vi "Actor Core.vi"(8 "error in":errorcluster caption="错误输入", 11 "DialogueM in":refnum<class "DialogueM.lvclass"> caption="操作者输入") -> (0 "error out":errorcluster caption="错误输出", 3 "Actor out":refnum<class "Actor.lvclass"> caption="操作者输出")   [LabVIEW 2014, in "DialogueManagement.lvlib" / "DialogueM.lvclass"]
doc: "(<B>文件名</B>：Actor Framework.lvlib:Actor.lvclass:Actor Core.vi)\n\n接收发送至操作者的消息，响应消息并处理可能导致操作者关闭的错误。\n\n子孙类重写该VI，使操作者完成特定的任务。使用调用父方法节点实现重写。"
uses:
  DialogueM.lvclass
  <vilib>/ActorFramework/Actor/Actor.lvclass
  <vilib>/ActorFramework/Actor/Actor.lvclass/Actor.ctl
  DialogueM.lvclass/DialogueM.ctl
  <vilib>/ActorFramework/Message Enqueuer/Message Enqueuer.lvclass/Message Enqueuer.ctl
  <vilib>/ActorFramework/Message Enqueuer/Enqueue.vi
  <vilib>/ActorFramework/Message Priority Queue/Priority Enqueue.vi
panel:
  out "Actor out 2":refnum<class "Actor.lvclass"> caption="操作者输出"
  out "语音信号输出字符串 2":string
  in  "停止信号":bool
  out "系统回应 4":string caption="标准输出"
  out "CM #":i32=-1
  out "InstructionIn":string
  out "系统回应 3":string caption="标准输出"
  out "系统回应 2":string caption="标准输出"
  out "格式化机器人指令":string[][](array[string])
  out "系统回应":string caption="标准输出"
  in  "重来":bool
  out "显示窗口":string
  out "语音信号输出字符串":string
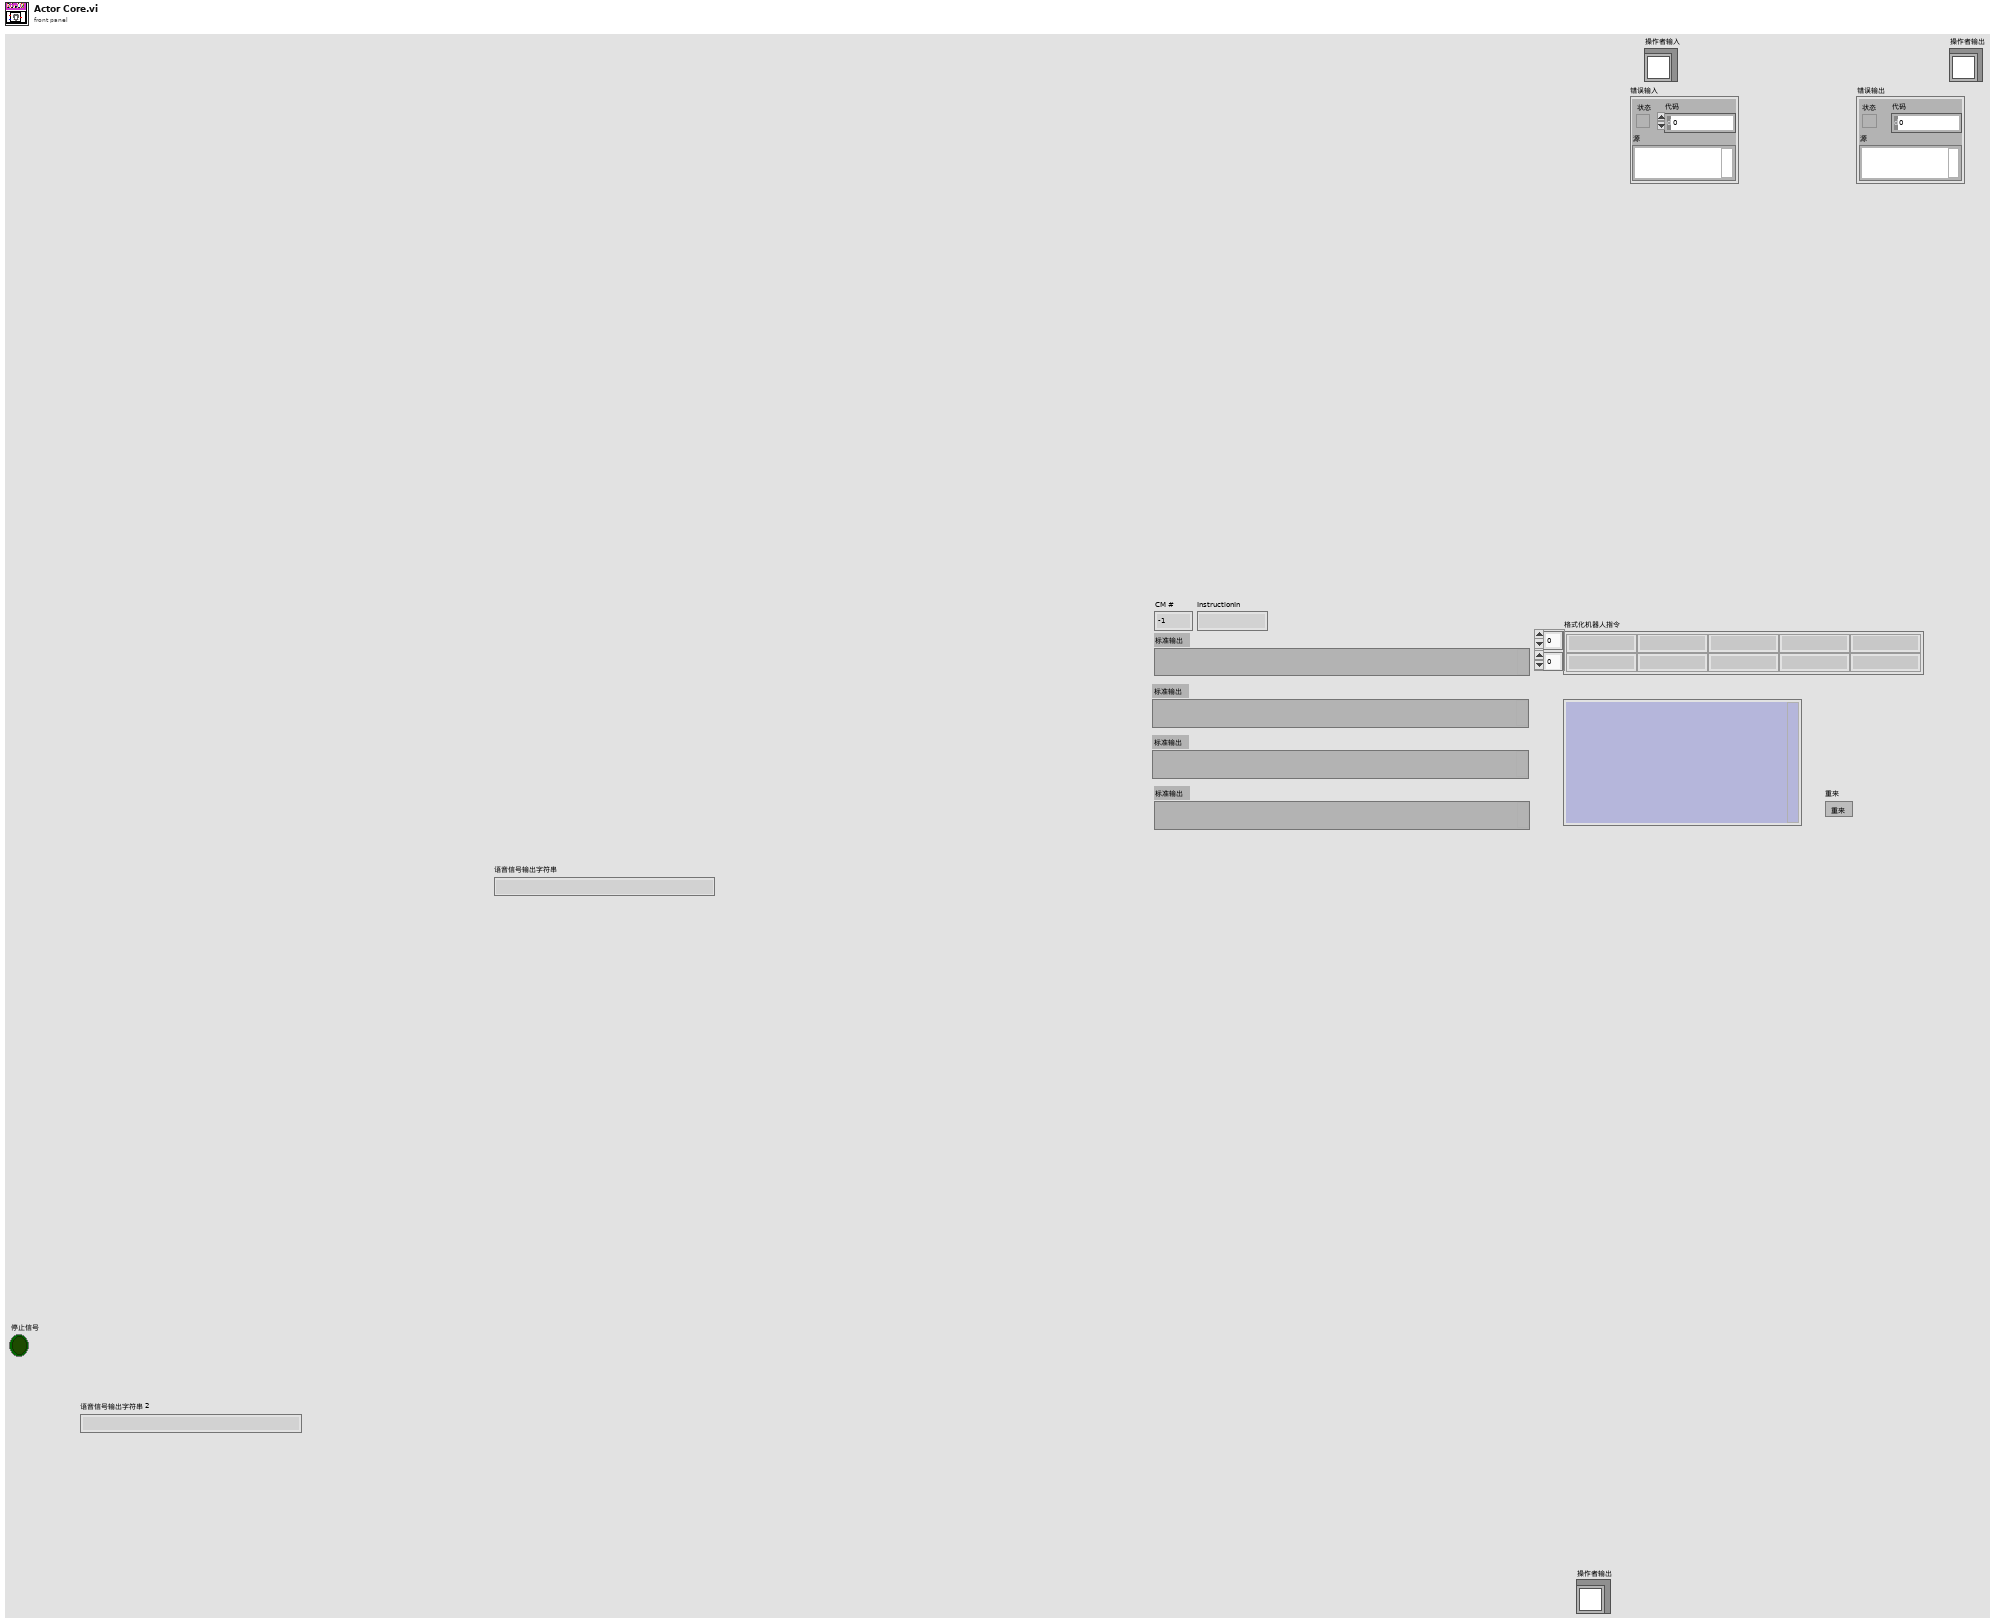
[diagram p1: front panel]
types:
  T1 = cluster{"输出数组":string[][], "CM #":i32, i32, string}
  T2 = cluster{"Stop":refnum<user-event>, "Text":refnum<user-event>, "Connected":refnum<user-event>}
  T3 = enum16{"open", "replace", "create", "open or create", "replace or create", "replace or create with confirmation"}
  T4 = cluster{"输出数组":string[][], "CM #":i32, "CM #":i32, string}
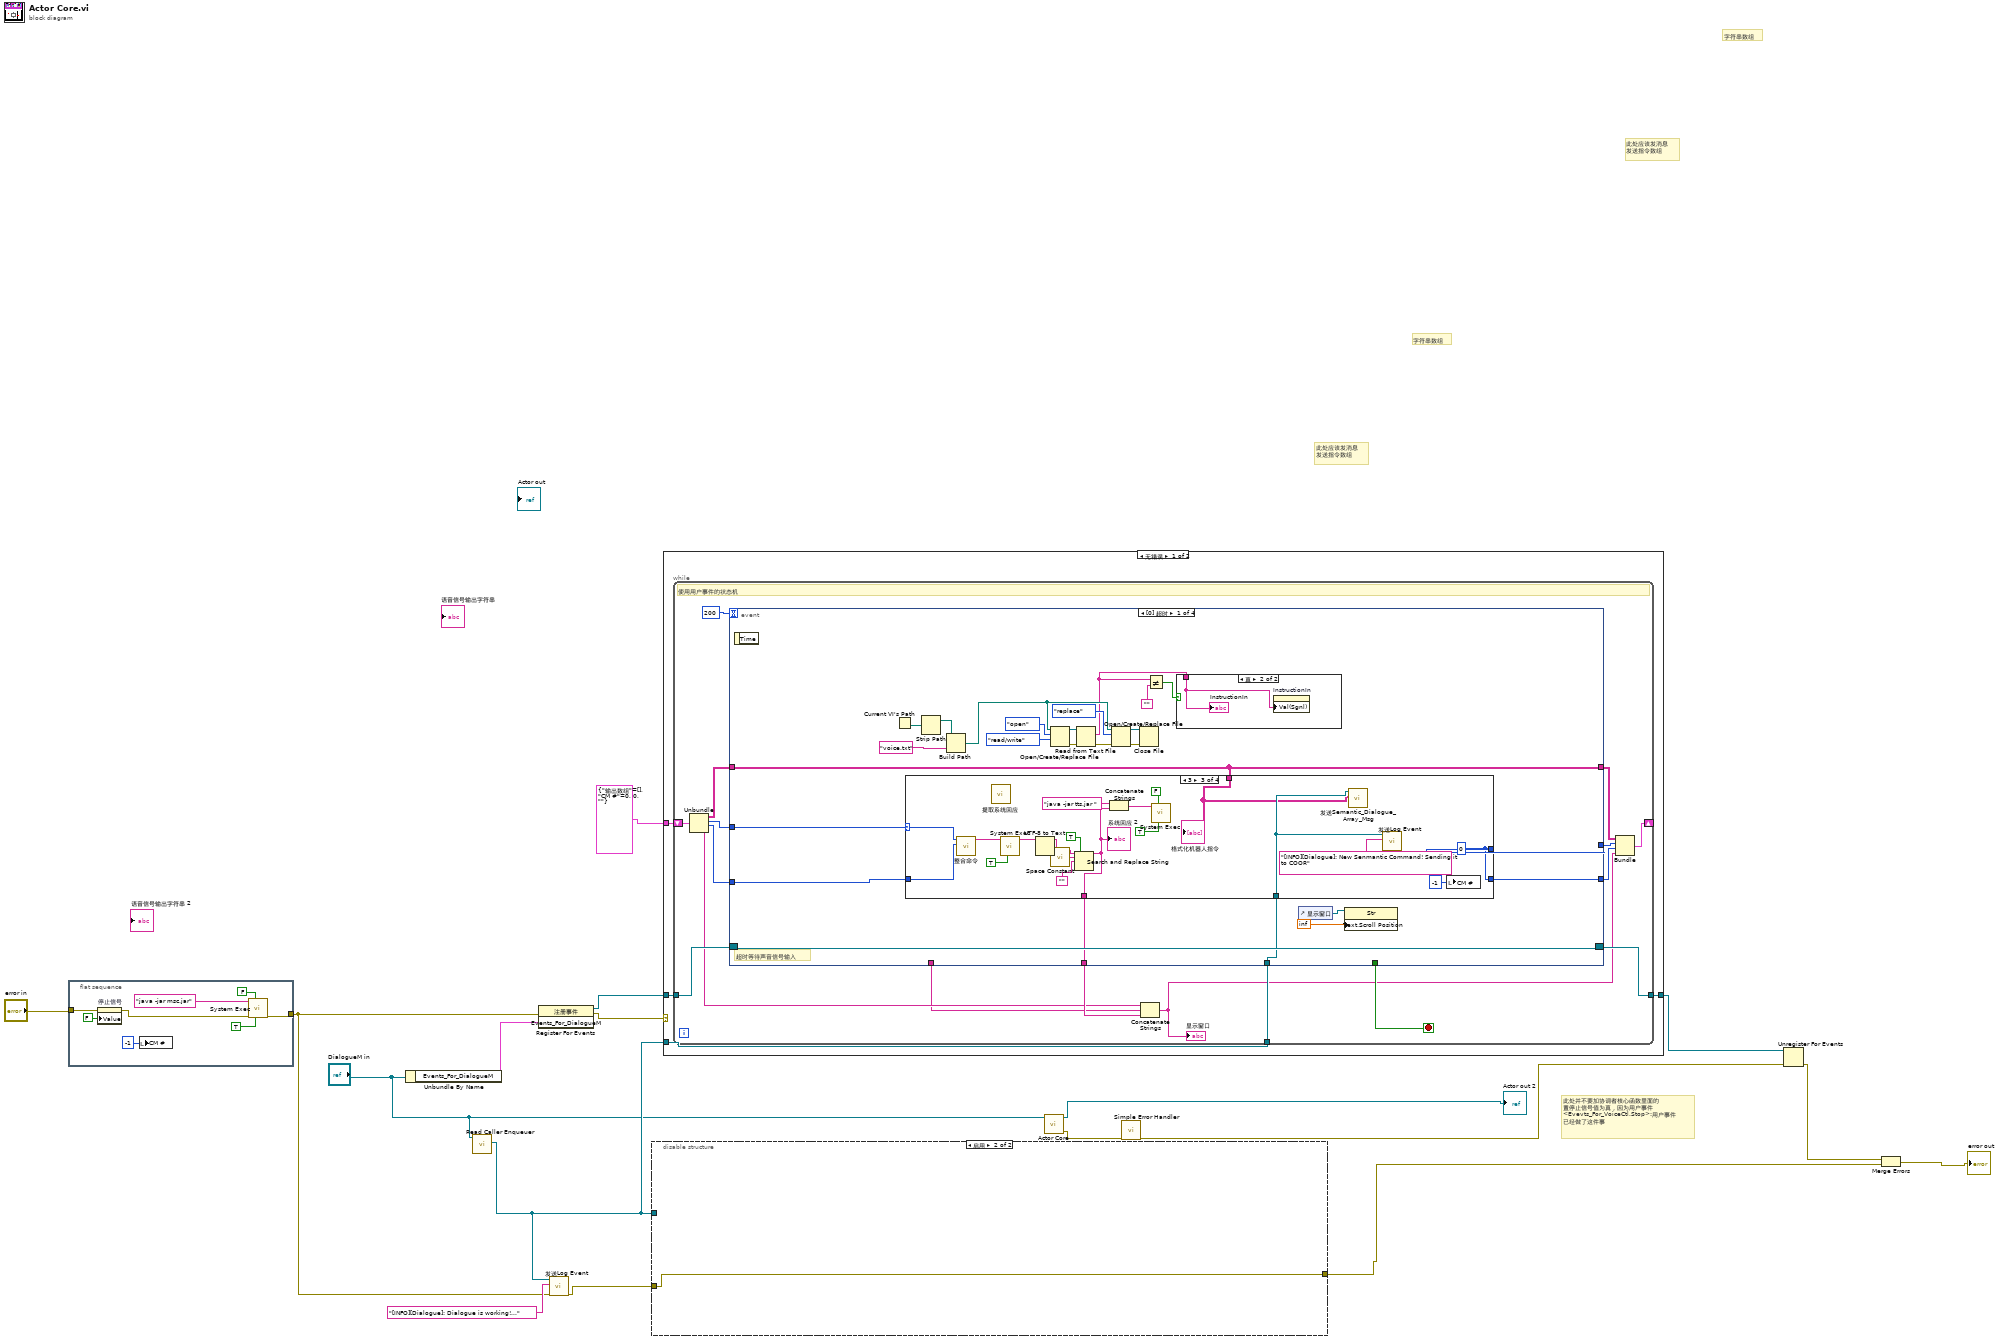
[diagram p0: block diagram]
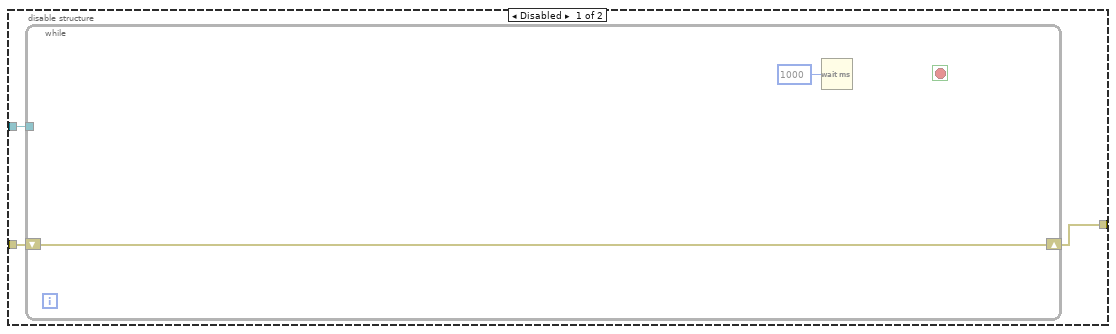
[diagram p2: hidden frame]
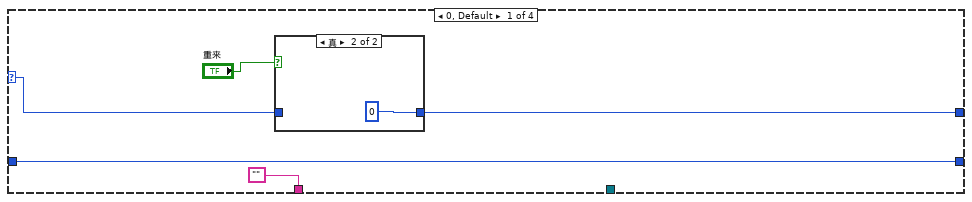
[diagram p3: hidden frame]
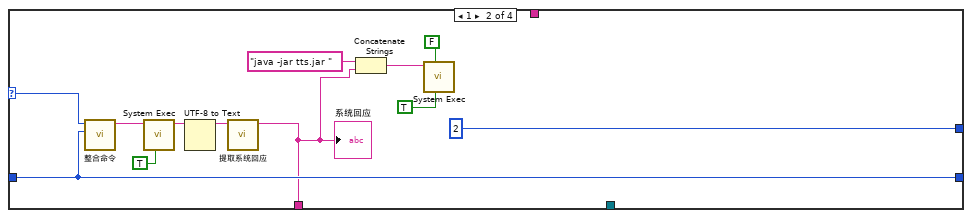
[diagram p5: hidden frame]
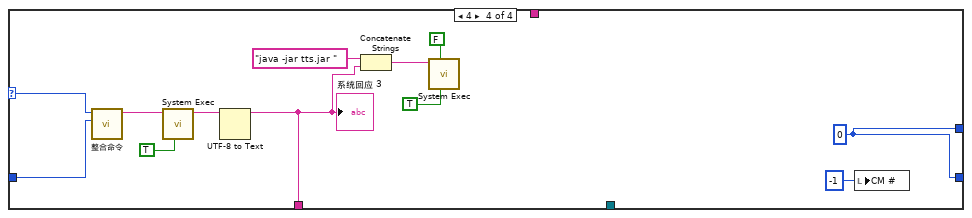
[diagram p6: hidden frame]
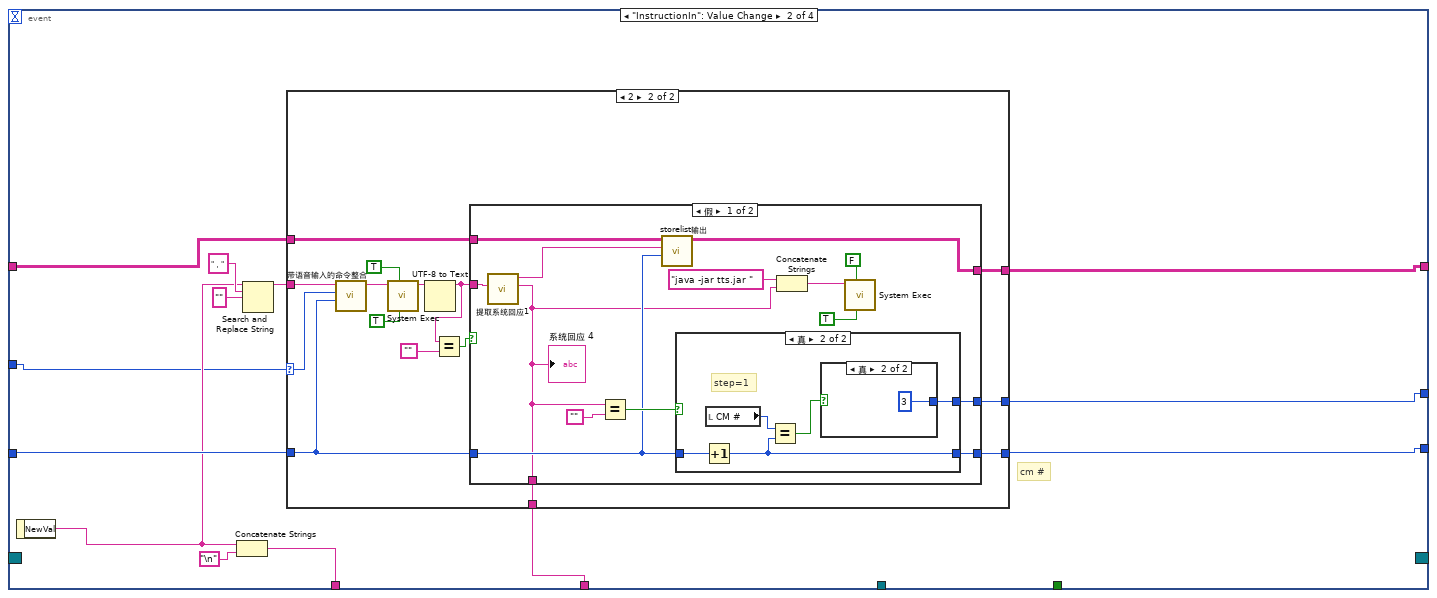
[diagram p8: hidden frame]
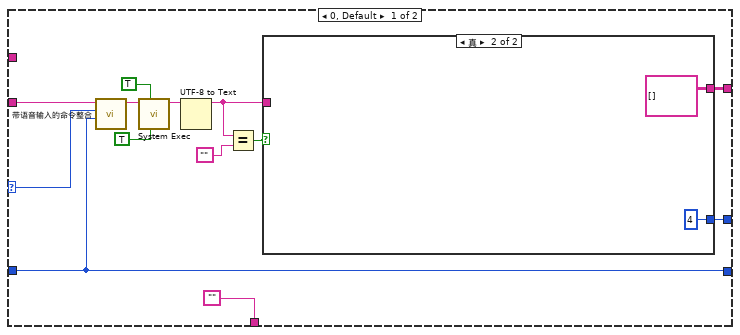
[diagram p9: hidden frame]
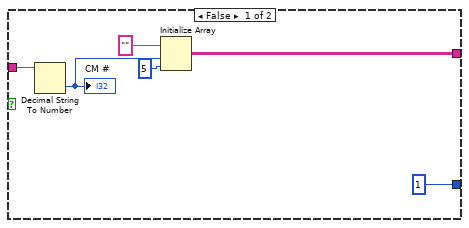
[diagram p10: hidden frame]
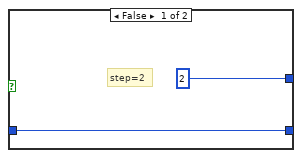
[diagram p11: hidden frame]
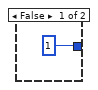
[diagram p12: hidden frame]
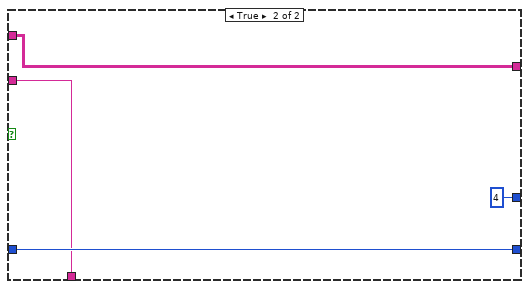
[diagram p13: hidden frame]
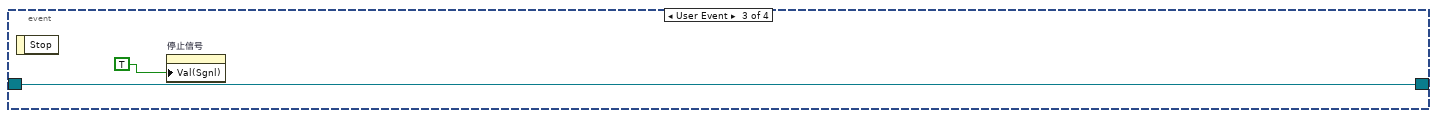
[diagram p14: hidden frame]
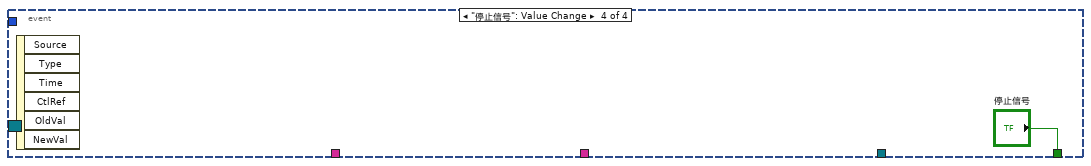
[diagram p15: hidden frame]
diagram:
  # "字符串数组"
  # "此处应该发消息\n发送指令数组"
  # "此处并不要加协调者核心函数里面的\n置停止信号值为真，因为用户事件\n<Evevts_For_VoiceCtl.Stop>:用户事件\n已经做了这件事"
  # "字符串数组"
  # "此处应该发消息\n发送指令数组"
  n1 = flat-sequence {
    tunnel: "error in" -> [w25]
    tunnel: [w19] -> w6
    frame #0 {
      n2 = property on="停止信号" class="Bool (严格)"(error in=w25, "Value"=FALSE ("停止信号")) -> (error out=w20:errorcluster)  [unwired: 1 in, 1 out]
      n3 = local write "CM #"(-1 ("CM #")) -> ()
      n4 = call <vilib>:"System Exec.vi"("run minimized? (F)"=TRUE, "wait until completion? (T)"=FALSE, "error in (no error)"=w20, "command line"="java -jar msc.jar") -> ("error out"=w19:errorcluster)  [unwired: 4 in, 3 out]
    }
  }
  n5 = Unbundle By Name("DialogueM in") -> ("Events_For_DialogueM"=w17:T2)
  n6 = call <vilib>:"Read Caller Enqueuer.vi"("Actor"="DialogueM in") -> ("Caller Enqueuer"=w9:refnum<class "Message Enqueuer.lvclass">)  [unwired: 10 in]
  n7 = register-events(error in=w6, w17) -> (reference out=w16:refnum<event-registration>, error out=w15:errorcluster)  [unwired: 1 in]
  n8 = call "发送Log Event.vi"("error in (no error)"=w6, "Event Text"="[INFO][Dialogue]: Dialogue is working!...", "消息待入队列"=w9) -> ("error out"=w10:cluster{"状态":bool, "代码":i32, "源":string})  [unwired: 7 in, 1 out]
  n9 = disable-structure shown="启用" {
    disable-tunnel: w10 -> [w28 w31]
    disable-tunnel: w9 -> [w27 _]
    disable-tunnel: [w26 w31] -> w5
    frame Disabled {
      n10 = while {
        tunnel: w27 -> [_]
        shift-right: [w29] -> w26
        shift-left: w28 -> [w29]
        stop <- _ stop-if-true
        n11 = Wait (ms)(milliseconds to wait=u32 1000 ("等待时间（毫秒）")) -> ()  [unwired: 1 out]
      }
    }
    frame Enabled {
    }
  }
  n12 = case shown="无错误" w15 {
    tunnel: [w35 w208] -> w12
    tunnel: w16 -> [w34 w208]
    tunnel: w9 -> [w33 _]
    tunnel: T1 {"输出数组"=[], "CM #"=0, 0, ""} -> [w32 _]
    frame No Error {
      n13 = while {
        tunnel: [w51] -> w35
        tunnel: w34 -> [w50]
        tunnel: w33 -> [w49]
        shift-right: [w39] -> _
        shift-left: w32 -> [w47]
        stop <- w52 stop-if-true
        # "使用用户事件的状态机"
        n14 = Unbundle(w47) -> ("输出数组"=w40:string[][], "CM #"=w41:i32, w42:i32, w37:string)
        n15 = event shown="[0] 超时" {
          selector: w50 -> [w77 _ w206 _]
          dyn-events: [w77 _ w206 _] -> w51
          timeout: 200 -> [_ _ _ _]
          tunnel: [_ _ _ "停止信号"] -> w52
          tunnel: w49 -> [w55 _ _ _]
          tunnel: w40 -> [w56 w132 _ _]
          tunnel: w41 -> [w61 w130 _ _]
          tunnel: w42 -> [w60 w134 _ _]
          tunnel: [w59 w129 _ _] -> w43
          tunnel: [w56 w137 _ _] -> w46
          tunnel: [w58 w136 _ _] -> w45
          tunnel: [w57 w135 _ _] -> w44
          tunnel: [_ w131 _ _] -> w36
          event Timeout {
            # "超时等待声音信号输入"
            n16 = event-data() -> ()  [unwired: 1 in, 1 out]
            n17 = Current VI's Path() -> (path=w76:path)
            n18 = case shown="3" w61 {
              selector: w61 -> [w78 w92 w113 w125]
              tunnel: [w79 2 w105 w117] -> w58
              tunnel: w60 -> [w81 w90 w111 w123]
              tunnel: ["" w85 w97 w118] -> w59
              tunnel: [w81 w90 w105 w117] -> w57
              tunnel: w56 -> [_ _ w102 _]
              tunnel: w55 -> [_ _ w103 _]
              frame 0, Default {
                n19 = case shown="真" "重来" {
                  tunnel: [w83 0] -> w79
                  tunnel: w78 -> [w83 _]
                  frame False {
                  }
                  frame True {
                  }
                }
              }
              frame 1 {
                n20 = call "整合命令.vi"("CM"=w90, "step"=w92) -> ("命令"=w91:string)  [unwired: 9 in]
                n21 = call <vilib>:"System Exec.vi"("run minimized? (F)"=TRUE, "command line"=w91) -> ("standard output"=w95:string)  [unwired: 6 in, 3 out]
                n22 = UTF-8 to Text(11:w95) -> (3:w94:string)  [unwired: 2 in, 1 out]
                n23 = call "提取系统回应.vi"("字符串"=w94) -> ("系统回应"=w85:string)  [unwired: 10 in]
                "系统回应" <- w85
                n24 = Concatenate Strings("java -jar tts.jar " ("command line"), w85) -> (w89:string)
                n25 = call <vilib>:"System Exec.vi"("run minimized? (F)"=TRUE, "wait until completion? (T)"=FALSE, "command line"=w89) -> ()  [unwired: 5 in, 4 out]
              }
              frame 3 {
                w105 = 0 ("CM #")
                n26 = call "整合命令.vi"("CM"=w111, "step"=w113) -> ("命令"=w112:string)  [unwired: 9 in]
                n27 = call "提取系统回应.vi"() -> ()  [unwired: 11 in, 1 out]
                n28 = call <vilib>:"System Exec.vi"("run minimized? (F)"=TRUE, "command line"=w112) -> ("standard output"=w115:string)  [unwired: 6 in, 3 out]
                n29 = UTF-8 to Text(11:w115) -> (3:w98:string)  [unwired: 2 in, 1 out]
                n30 = call <vilib>:"Space Constant.vi"() -> ("String"=w101:string)
                n31 = Search and Replace String(replace all?=TRUE ("替换全部？(F)"), input string=w98, search string=w101, replace string="") -> (result string=w97:string)  [unwired: 4 in, 3 out]
                "系统回应 2" <- w97
                n32 = Concatenate Strings("java -jar tts.jar " ("command line"), w97) -> (w110:string)
                n33 = call <vilib>:"System Exec.vi"("run minimized? (F)"=TRUE, "wait until completion? (T)"=FALSE, "command line"=w110) -> ()  [unwired: 5 in, 4 out]
                n34 = call "发送Semantic_Dialogue_Array_Msg.vi"("值(信号)"=w102, "消息待入队列"=w103) -> ()  [unwired: 8 in, 2 out]
                n35 = call "发送Log Event.vi"("Event Text"="[INFO][Dialogue]: New Senmantic Command! Sending it to COOR", "消息待入队列"=w103) -> ()  [unwired: 8 in, 2 out]
                n36 = local write "CM #"(-1 ("CM #")) -> ()
                "格式化机器人指令" <- w102
              }
              frame 4 {
                w117 = 0 ("CM #")
                n37 = call "整合命令.vi"("CM"=w123, "step"=w125) -> ("命令"=w124:string)  [unwired: 9 in]
                n38 = call <vilib>:"System Exec.vi"("run minimized? (F)"=TRUE, "command line"=w124) -> ("standard output"=w127:string)  [unwired: 6 in, 3 out]
                n39 = UTF-8 to Text(11:w127) -> (3:w118:string)  [unwired: 2 in, 1 out]
                "系统回应 3" <- w118
                n40 = Concatenate Strings("java -jar tts.jar " ("command line"), w118) -> (w122:string)
                n41 = call <vilib>:"System Exec.vi"("run minimized? (F)"=TRUE, "wait until completion? (T)"=FALSE, "command line"=w122) -> ()  [unwired: 5 in, 4 out]
                n42 = local write "CM #"(-1 ("CM #")) -> ()
              }
            }
            n43 = Strip Path(path=w76) -> (stripped path=w73:path)  [unwired: 1 out]
            n44 = Build Path(base path=w73, name or relative path="voice.txt" ("名称或相对路径")) -> (appended path=w75:path)
            n45 = Open/Create/Replace File(file path (use dialog)=w75, operation (0:open)=T3."open" ("操作(0:open)"), access (0:read/write)=enum16{"read/write", "read-only", "write-only"}."read/write" ("权限(0:read/write)")) -> (refnum out=w68:refnum<file>, error out=w67:errorcluster)  [unwired: 3 in, 1 out]
            n46 = Read from Text File(file (use dialog)=w68, error in=w67) -> (text=w62:string, error out=w70:errorcluster)  [unwired: 2 in, 2 out]
            n47 = Open/Create/Replace File(file path (use dialog)=w75, error in=w70, operation (0:open)=T3."replace" ("操作(0:open)")) -> (refnum out=w71:refnum<file>, error out=w72:errorcluster)  [unwired: 3 in, 1 out]
            n48 = Close File(refnum=w71, error in=w72) -> ()  [unwired: 2 out]
            n49 = Not Equal?(x=w62, y="") -> (x != y?=w63:bool)
            n50 = case shown="真" w63 {
              tunnel: w62 -> [_ w128]
              frame False {
              }
              frame True {
                n51 = property on="InstructionIn" class="Str"("Val(Sgnl)"=w128) -> ()  [unwired: 2 in, 2 out]
                "InstructionIn" <- w128
              }
            }
            n52 = control-ref of="显示窗口"() -> (w54:refnum<vi>)
            n53 = property on="属性节点" class="Str"(reference=w54, "Text.Scroll Position"=inf) -> ()  [unwired: 1 in, 2 out]
          }
          event "InstructionIn": Value Change {
            # "cm #"
            n54 = event-data() -> ("NewVal"=w133:string)  [unwired: 1 in]
            n55 = Concatenate Strings(w133, "\n") -> (w131:string)
            n56 = Search and Replace String(input string=w133, search string="，" ("子字符串(\"\")"), replace string="" ("替换字符串(\"\")")) -> (result string=w138:string)  [unwired: 5 in, 3 out]
            n57 = case shown="2" w130 {
              selector: w130 -> [w149 w171]
              tunnel: [w148 w175] -> w135
              tunnel: w134 -> [w148 w168]
              tunnel: [w152 w174] -> w136
              tunnel: ["" w169] -> w129
              tunnel: w138 -> [w147 w172]
              tunnel: [w145 w166] -> w137
              tunnel: w132 -> [_ w167]
              frame 0, Default {
                n58 = call "带语音输入的命令整合.vi"("CM"=w148, "step"=w149, "输入指令"=w147) -> ("命令"=w146:string)  [unwired: 8 in]
                n59 = call <vilib>:"System Exec.vi"("run minimized? (F)"=TRUE, "wait until completion? (T)"=TRUE, "command line"=w146) -> ("standard output"=w153:string)  [unwired: 5 in, 3 out]
                n60 = UTF-8 to Text(11:w153) -> (3:w143:string)  [unwired: 2 in, 1 out]
                n61 = Equal?(x=w143, y="") -> (x = y?=w142:bool)
                n62 = case shown="真" w142 {
                  tunnel: [1 4] -> w152
                  tunnel: w143 -> [w159 _]
                  tunnel: [w155 string[][] []] -> w145
                  frame False {
                    n63 = Decimal String To Number(string=w159) -> (number=w157:i32)  [unwired: 2 in, 1 out]
                    "CM #" <- w157
                    n64 = Initialize Array("", w157, 5 ("维数大小")) -> (w155:string[][])
                  }
                  frame True {
                  }
                }
              }
              frame 2 {
                n65 = call "带语音输入的命令整合.vi"("CM"=w168, "step"=w171, "输入指令"=w172) -> ("命令"=w170:string)  [unwired: 8 in]
                n66 = call <vilib>:"System Exec.vi"("run minimized? (F)"=TRUE, "wait until completion? (T)"=TRUE, "command line"=w170) -> ("standard output"=w176:string)  [unwired: 5 in, 3 out]
                n67 = UTF-8 to Text(11:w176) -> (3:w164:string)  [unwired: 2 in, 1 out]
                n68 = Equal?(x=w164, y="") -> (x = y?=w163:bool)
                n69 = case shown="假" w163 {
                  tunnel: [w189 w204] -> w175
                  tunnel: [w188 4] -> w174
                  tunnel: w164 -> [w187 w201]
                  tunnel: [w178 w201] -> w169
                  tunnel: w168 -> [w185 w204]
                  tunnel: w167 -> [w184 w202]
                  tunnel: [w183 w202] -> w166
                  frame False {
                    n70 = call "提取系统回应1.vi"("字符串"=w187) -> ("系统回应"=w178:string, "子字符串之前"=w186:string)  [unwired: 9 in]
                    "系统回应 4" <- w178
                    n71 = Equal?(x=w178, y="") -> (x = y?=w190:bool)
                    n72 = call "storelist输出.vi"("CM"=w185, 10:"storelist"=w186, 11:"storelist"=w184) -> ("输出数组"=w183:string[][])  [unwired: 8 in]
                    n73 = case shown="真" w190 {
                      tunnel: [2 w197] -> w188
                      tunnel: w185 -> [w193 w198]
                      tunnel: [w193 w194] -> w189
                      frame False {
                        # "step=2"
                      }
                      frame True {
                        # "step=1"
                        n74 = Increment(x=w198) -> (x+1=w194:i32)
                        n75 = local read "CM #"() -> (w196:i32)
                        n76 = Equal?(x=w196, y=w194) -> (x = y?=w195:bool)
                        n77 = case shown="真" w195 {
                          tunnel: [1 3] -> w197
                          frame False {
                          }
                          frame True {
                          }
                        }
                      }
                    }
                    n78 = Concatenate Strings("java -jar tts.jar " ("command line"), w178) -> (w182:string)
                    n79 = call <vilib>:"System Exec.vi"("run minimized? (F)"=TRUE, "wait until completion? (T)"=FALSE, "command line"=w182) -> ()  [unwired: 5 in, 4 out]
                  }
                  frame True {
                  }
                }
              }
            }
          }
          event User Event {
            n80 = event-data() -> ()  [unwired: 1 in, 1 out]
            n81 = property on="停止信号" class="Bool (严格)"("Val(Sgnl)"=TRUE) -> ()  [unwired: 2 in, 2 out]
          }
          event "停止信号": Value Change {
            n82 = event-data() -> ()  [unwired: 1 in, 6 out]
          }
        }
        n83 = Concatenate Strings(w37, w36, w43) -> (w38:string)
        "显示窗口" <- w38
        n84 = Bundle("输出数组"=w46, "CM #"=w45, "CM #"=w44, w38) -> (w39:T4)  [unwired: 1 in]
      }
    }
    frame Error {
    }
  }
  n85 = call-parent "Actor Core.vi"("Actor in"="DialogueM in") -> ("error out"=w14:errorcluster, "Actor out"=→"Actor out 2":refnum<class "Actor.lvclass">)  [unwired: 9 in]
  n86 = call <vilib>:"Simple Error Handler.vi"("error in (no error)"=w14) -> ("error out"=w13:errorcluster)  [unwired: 4 in, 4 out]
  n87 = Unregister For Events(event registration refnum=w12, error in=w13) -> (error out=w11:errorcluster)
  n88 = Merge Errors(w11, w5) -> (→"error out":errorcluster)
